vi "3.5.vi"() -> ()   [LabVIEW 2014]
panel:
  out "Warning Y/N":bool
  out "Warning Text":string
  in  "Min Temp":dbl
  in  "Max Temp":dbl
  in  "Current Temp":dbl
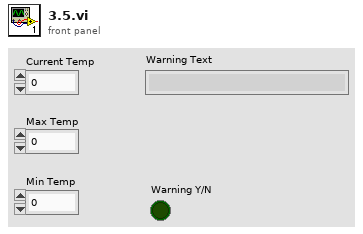
[diagram p1: front panel]
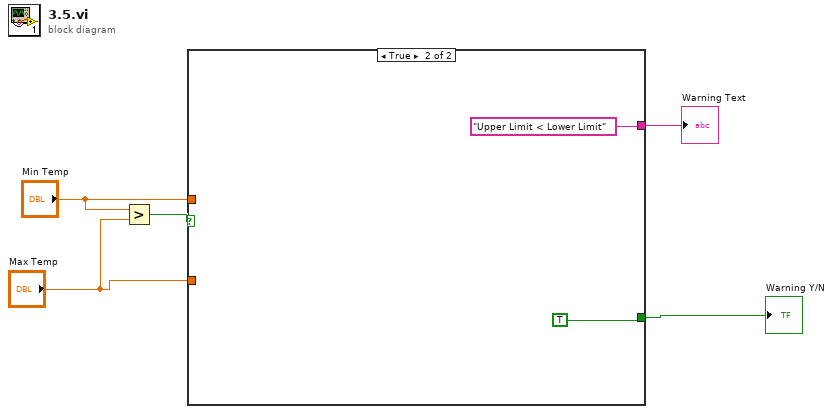
[diagram p0: block diagram]
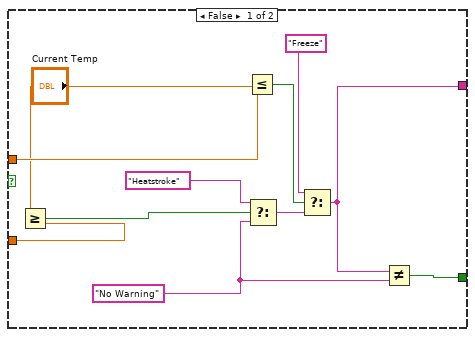
[diagram p2: hidden frame]
diagram:
  n1 = Greater?(x="Min Temp", y="Max Temp") -> (0:w2:bool)
  n2 = case shown="True" w2 {
    tunnel: [w12 "Upper Limit < Lower Limit"] -> w5
    tunnel: [w6 TRUE] -> w4
    tunnel: "Max Temp" -> [w9 _]
    tunnel: "Min Temp" -> [w8 _]
    frame False {
      w11 = "No Warning"
      n3 = Greater Or Equal?(x="Current Temp", y=w9) -> (x >= y?=w10:bool)
      n4 = Less Or Equal?(x="Current Temp", y=w8) -> (x <= y?=w16:bool)
      n5 = Select(t="Heatstroke", s=w10, f=w11) -> (s? t:f=w13:string)
      n6 = Select(t="Freeze", s=w16, f=w13) -> (s? t:f=w12:string)
      n7 = Not Equal?(x=w12, y=w11) -> (x != y?=w6:bool)
    }
    frame True {
    }
  }
  "Warning Text" <- w5
  "Warning Y/N" <- w4
